vi "runtest Auto Increment User Prefix Field.vi"(3 "Field Value":string) -> (1 "New Field Value":string)   [LabVIEW 2011]
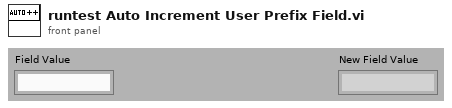
[diagram p1: front panel]
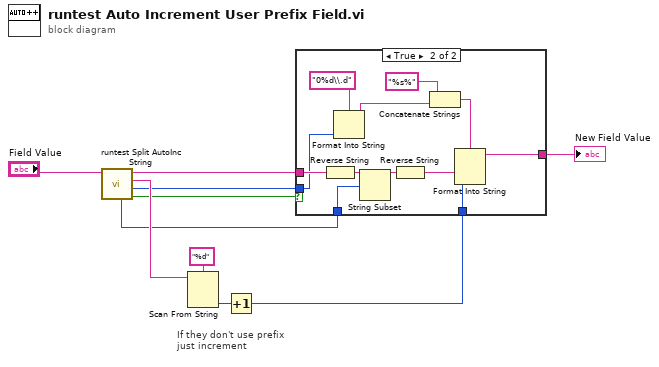
[diagram p0: block diagram]
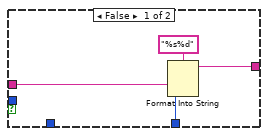
[diagram p2: hidden frame]
diagram:
  # "If they don't use prefix\njust increment"
  n1 = call "runtest Split AutoInc String.vi"("Auto Inc Field Value"="Field Value") -> ("Use zero width?"=w4:bool, "Width"=w5:i32, "Increment Value"=w10:string, "Auto Inc Field Prefix"=w6:string, "# Preceding zeros"=w1:i32)  [unwired: 6 out]
  n2 = Scan From String(format string="%d", input string=w10) -> (output 1=w7:i32)  [unwired: 2 in, 4 out]
  n3 = Increment(x=w7) -> (x+1=w3:i32)
  n4 = case shown="True" w4 {
    tunnel: w3 -> [w13 w26]
    tunnel: w6 -> [w12 w20]
    tunnel: [w11 w25] -> w2
    tunnel: w5 -> [_ w16]
    tunnel: w1 -> [_ w15]
    frame False {
      n5 = Format Into String(format string="%s%d", w12, w13) -> (resulting string=w11:string)  [unwired: 2 in, 1 out]
    }
    frame True {
      n6 = Reverse String(1:w20) -> (0:w19:string)
      n7 = Format Into String(format string="0%d\\.d", w16) -> (resulting string=w22:string)  [unwired: 2 in, 1 out]
      n8 = String Subset(string=w19, offset (0)=w15) -> (substring=w18:string)  [unwired: 1 out]
      n9 = Reverse String(1:w18) -> (0:w17:string)
      n10 = Concatenate Strings("%s%" ("format string"), w22) -> (w21:string)
      n11 = Format Into String(format string=w21, w17, w26) -> (resulting string=w25:string)  [unwired: 2 in, 1 out]
    }
  }
  "New Field Value" <- w2
